vi "_PassAllowedMessage - Mapping.vi"(5 "Mapping":cluster{"broadcast":string, "API":string}[](array[cluster]), 8 "JKISM External Event":string) -> (2 "States":string)   [LabVIEW 2017, in "_csmlite.lvlib"]
uses:
  _csmlite.lvlib
  Communicable State Machine.lvlib
  _Shared/CSM Shared.lvlib
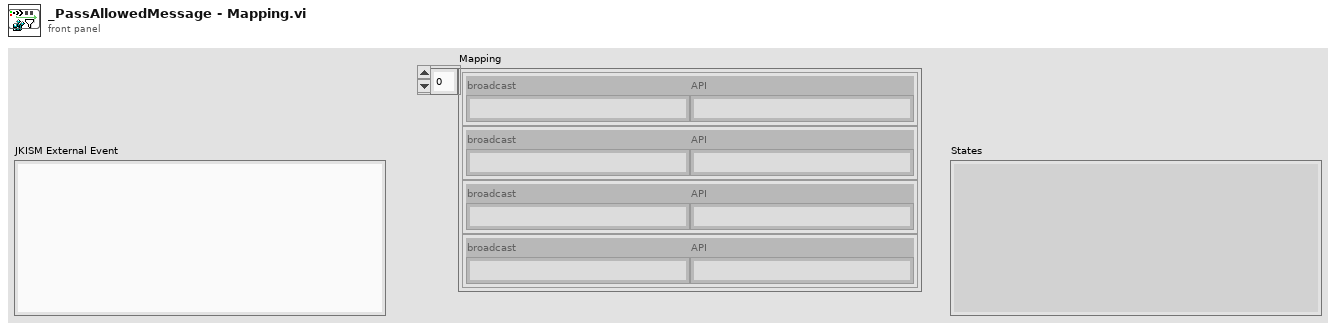
[diagram p1: front panel]
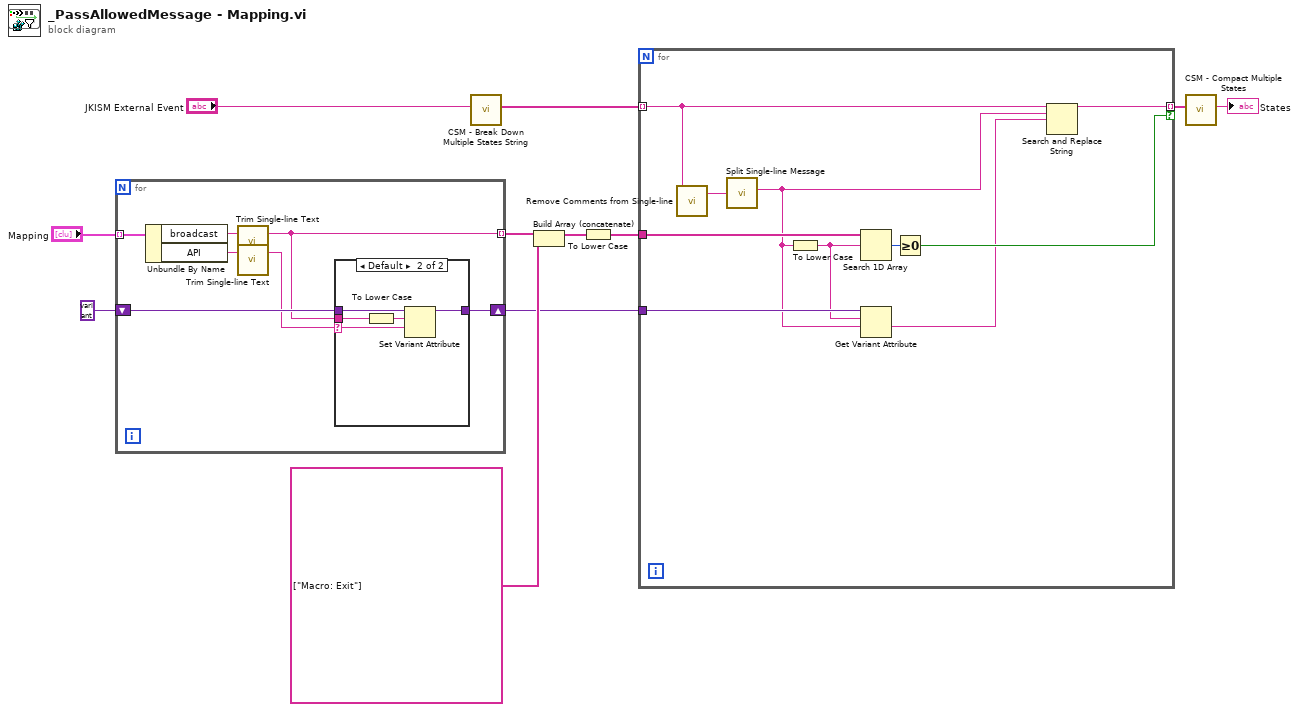
[diagram p0: block diagram]
diagram:
  n1 = for {
    tunnel: "Mapping" -> [w18] mode=indexing
    tunnel: [w12] -> w4 mode=indexing
    shift-right: [w16] -> w1
    shift-left: variant ("variant") -> [w17]
    n2 = Unbundle By Name(w18) -> ("broadcast"=w15:string, "API"=w14:string)
    n3 = call "Trim Single-line Text.vi"("single-line text"=w15) -> ("trimed text"=w12:string)  [unwired: 2 in]
    n4 = call "Trim Single-line Text.vi"("single-line text"=w14) -> ("trimed text"=w13:string)  [unwired: 2 in]
    n5 = case shown="Default" w13 {
      selector: w13 -> [_ w21]
      tunnel: w17 -> [w19 w24]
      tunnel: [w19 w23] -> w16
      tunnel: w12 -> [_ w20]
      frame "False" {
      }
      frame Default {
        n6 = To Lower Case(string=w20) -> (all lower case string=w22:string)
        n7 = Set Variant Attribute(Variant=w24, name=w22, value=w21) -> (Variant out=w23:variant)  [unwired: 1 in, 2 out]
      }
    }
  }
  n8 = call "CSM - Break Down Multiple States String.vi"("States"="JKISM External Event") -> ("Multiple States"=w8:string[])  [unwired: 10 in]
  n9 = Build Array (concatenate)(w4, string[] ["Macro: Exit"] ("element")) -> (w7:string[])
  n10 = To Lower Case(string=w7) -> (all lower case string=w6:string[])
  n11 = for {
    tunnel: w8 -> [w27] mode=indexing
    tunnel: [w28] -> w9 mode=indexing if=w31
    tunnel: w6 -> [w33]
    tunnel: w1 -> [w30]
    n12 = call "Remove Comments from Single-line.vi"("single-line text"=w27) -> ("single-line text without comments"=w34:string)  [unwired: 2 in]
    n13 = call "Split Single-line Message.vi"("single-line text"=w34) -> ("state"=w26:string)  [unwired: 6 in, 3 out]
    n14 = To Lower Case(string=w26) -> (all lower case string=w29:string)
    n15 = Search 1D Array(1D array=w33, element=w29) -> (index of element=w32:i32)  [unwired: 1 in]
    n16 = Get Variant Attribute(Variant=w30, name=w29, default value (empty Variant)=w26) -> (value=w25:string)  [unwired: 1 in, 3 out]
    n17 = Greater Or Equal To 0?(x=w32) -> (x >= 0?=w31:bool)
    n18 = Search and Replace String(input string=w27, search string=w26, replace string=w25) -> (result string=w28:string)  [unwired: 5 in, 3 out]
  }
  n19 = call "CSM - Compact Multiple States.vi"("Multiple States"=w9) -> ("States"=→"States":string)  [unwired: 9 in]
